vi "Get Cal Coeff.vi"(0 "instrument handle":refnum<k15>="PXI1Slot2", 7 "Correction Factor":T1(ring), 11 "Error In":errorcluster) -> (4 "instrument handle out":refnum<k15>="PXI1Slot2", 8 "Correction Factor Array":csg[](array[numeric]), 15 "Error Out":errorcluster)   [LabVIEW 2013]
uses:
  niVNAAn_CDll.dll
  niVNA.dll
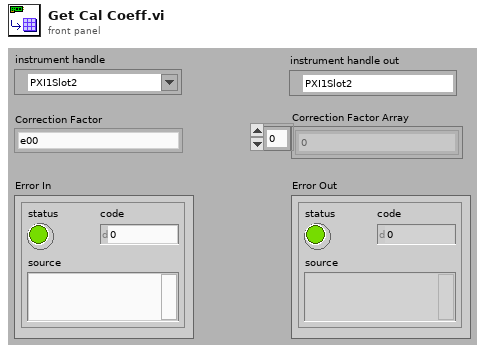
[diagram p1: front panel]
types:
  T1 = enum16{"e00", "e11", "e10e01", "e10e32", "e22", "e30", "e'33", "e'22", "e'23e'32", "e'23e'01", "e'11", "e'03"}
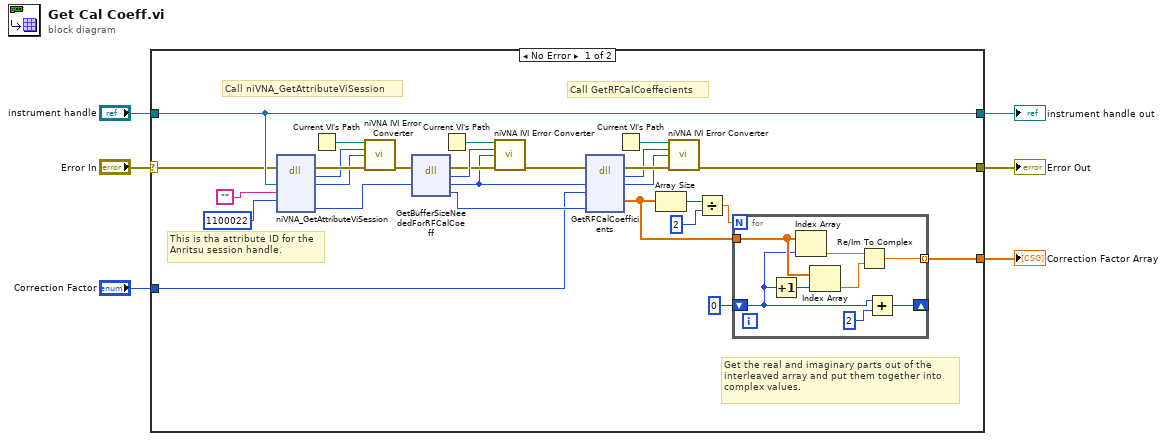
[diagram p0: block diagram]
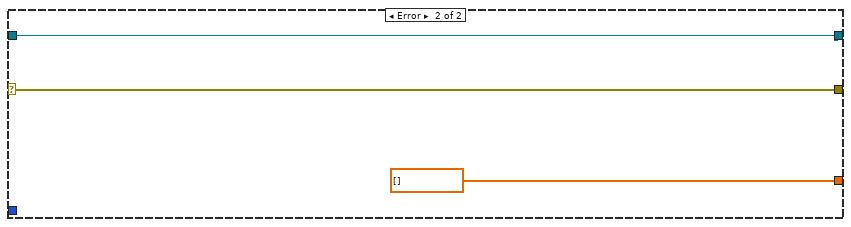
[diagram p2: hidden frame]
diagram:
  n1 = case shown="No Error" "Error In" {
    selector: "Error In" -> [w7 w44]
    tunnel: [w12 csg[] []] -> w6
    tunnel: "Correction Factor" -> [w11 _]
    tunnel: "instrument handle" -> [w8 w45]
    tunnel: [w9 w44] -> w4
    tunnel: [w8 w45] -> w2
    frame No Error {
      # "This is tha attribute ID for the\nAnritsu session handle."
      # "Get the real and imaginary parts out of the\ninterleaved array and put them together into\ncomplex values."
      # "Call GetRFCalCoeffecients"
      # "Call niVNA_GetAttributeViSession"
      n2 = dll-call lib="niVNA**.*" fn="niVNA_GetAttributeViSession"(error in=w7, "instrumentHandle"=w8, "channel"="", "attributeID"=1100022) -> (error out=w29:errorcluster, "return type"=w28:i32, "instrumentHandle"=w27:i32, "value"=w20:i32)  [unwired: 5 in, 1 out]
      n3 = Current VI's Path() -> (path=w30:path)
      n4 = call <instrlib>:"niVNA IVI Error Converter.vi"("path to vi"=w30, "ivi error code"=w28, "instrument handle"=w27, "error in"=w29) -> ("error out"=w22:errorcluster)  [unwired: 11 out]
      n5 = dll-call lib="niVNAAn_CDll.dll" fn="GetBufferSizeNeededForRFCalCoeff"(error in=w22, "SessionId"=w20) -> (error out=w24:errorcluster, "return type"=w25:i32, "SessionId"=w19:i32, "arraySize"=w18:u32)  [unwired: 3 in, 1 out]
      n6 = Current VI's Path() -> (path=w23:path)
      n7 = call <instrlib>:"niVNA IVI Error Converter.vi"("path to vi"=w23, "ivi error code"=w25, "instrument handle"=w19, "error in"=w24) -> ("error out"=w21:errorcluster)  [unwired: 11 out]
      n8 = dll-call lib="niVNAAn_CDll.dll" fn="GetRFCalCoefficients"(error in=w21, "SessionId"=w19, "errorTerm"=w11, "readCount"=w18) -> (error out=w32:errorcluster, "return type"=w31:i32, "SessionId"=w26:i32, "coeff"=w16:sgl[])  [unwired: 5 in, 1 out]
      n9 = Current VI's Path() -> (path=w33:path)
      n10 = Array Size(array=w16) -> (size(s)=w15:i32)
      n11 = call <instrlib>:"niVNA IVI Error Converter.vi"("path to vi"=w33, "ivi error code"=w31, "instrument handle"=w26, "error in"=w32) -> ("error out"=w9:errorcluster)  [unwired: 11 out]
      n12 = Divide(x=w15, y=2) -> (x/y=w14:dbl)
      n13 = for {
        N: w14 -> [_]
        tunnel: w16 -> [w41]
        tunnel: [w38] -> w12 mode=indexing
        shift-right: [w37] -> _
        shift-left: 0 -> [w36]
        n14 = Increment(x=w36) -> (x+1=w42:i32)
        n15 = Index Array(array=w41, index=w36) -> (element=w39:sgl)
        n16 = Index Array(array=w41, index=w42) -> (element=w40:sgl)
        n17 = Re/Im To Complex(1:w40, 2:w39) -> (0:w38:csg)
        n18 = Add(x=w36, y=2) -> (x+y=w37:i32)
      }
    }
    frame Error {
    }
  }
  "instrument handle out" <- w2
  "Correction Factor Array" <- w6
  "Error Out" <- w4
